vi "ForceManualSwitches.vi"(9 "Switch Op":T4[](array[typedef]), 11 "output array 2":T1) -> (3 "output array 3":T1)   [LabVIEW 2014]
uses:
  Controls/SwitchOp.ctl
  Libraries/Map Data Folder/All-Lines.ctl
  Libraries/Map Data Folder/LineCluster.ctl
  Libraries/Map Data Folder/LineConnection.ctl
  Libraries/Map Data Folder/Map Data.lvlib
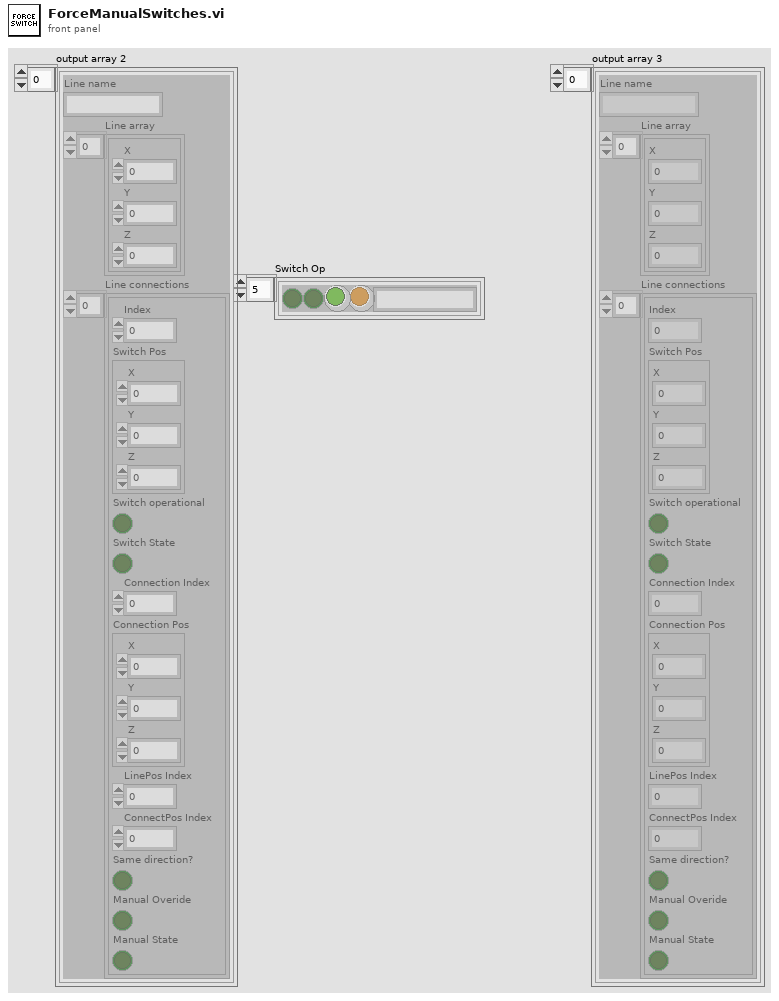
[diagram p1: front panel]
types:
  T1 = typedef "Map Data.lvlib/All-Lines.ctl" = T2[]
  T2 = typedef "Map Data.lvlib/LineCluster.ctl" = cluster{"Line name":string, "Line array":cluster{"X":dbl, "Y":dbl, "Z":dbl}[], "Line connections":T3[]}
  T3 = typedef "LineConnection.ctl" = cluster{"Index":i32, "Switch Pos":cluster{"X":dbl, "Y":dbl, "Z":dbl}, "Switch operational":bool, "Switch State":bool, "Connection Index":i32, "Connection Pos":cluster{"X":dbl, "Y":dbl, "Z":dbl}, "LinePos Index":i32, "ConnectPos Index":i32, "Same direction?":bool, "Manual Overide":bool, "Manual State":bool}
  T4 = typedef "SwitchOp.ctl" = cluster{"Switch operational":bool, "Switch State":bool, "Manual Overide":bool, "Manual State":bool, "Switch\nPosition":cluster{"X":dbl, "Y":dbl, "Z":dbl}, "Index":i32, "Connection Index":i32, "Switch Index":i32, string}
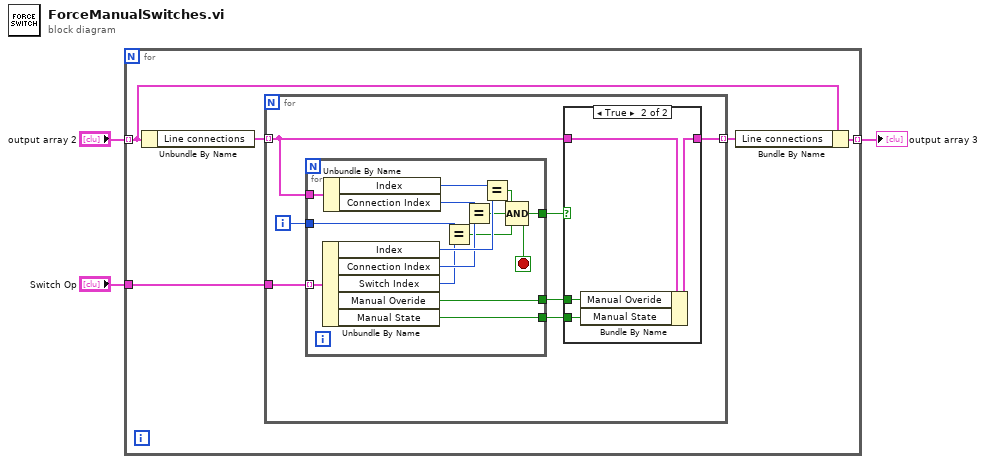
[diagram p0: block diagram]
diagram:
  n1 = for {
    tunnel: "output array 2" -> [w6] mode=indexing
    tunnel: "Switch Op" -> [w7]
    tunnel: [w4] -> w1 mode=indexing
    n2 = Unbundle By Name(w6) -> ("Line connections"=w8:T3[])
    n3 = for {
      tunnel: w8 -> [w12] mode=indexing
      tunnel: [w11] -> w5 mode=indexing
      tunnel: w7 -> [w15]
      i -> [w14]
      n4 = for {
        tunnel: w12 -> [w34]
        tunnel: w15 -> [w33] mode=indexing
        tunnel: w14 -> [w28]
        tunnel: [w23] -> w10
        tunnel: [w22] -> w9
        tunnel: [w21] -> w13
        stop <- w21 stop-if-true
        n5 = Unbundle By Name(w33) -> ("Index"=w32:i32, "Connection Index"=w29:i32, "Switch Index"=w27:i32, "Manual Overide"=w23:bool, "Manual State"=w22:bool)
        n6 = Unbundle By Name(w34) -> ("Index"=w31:i32, "Connection Index"=w30:i32)
        n7 = Equal?(x=w28, y=w27) -> (x = y?=w24:bool)
        n8 = Equal?(x=w30, y=w29) -> (x = y?=w25:bool)
        n9 = Equal?(x=w31, y=w32) -> (x = y?=w26:bool)
        n10 = Compound Arithmetic op=AND(w26, w25, w24) -> (w21:bool)
      }
      n11 = case shown="True" w13 {
        tunnel: w12 -> [w16 w20]
        tunnel: [w16 w19] -> w11
        tunnel: w10 -> [_ w18]
        tunnel: w9 -> [_ w17]
        frame False {
        }
        frame True {
          n12 = Bundle By Name(cluster=w20, "Manual Overide"=w18, "Manual State"=w17) -> (w19:T3)
        }
      }
    }
    n13 = Bundle By Name(cluster=w6, "Line connections"=w5) -> (w4:T2)
  }
  "output array 3" <- w1
